vi "FlatToRichrfcontrol_CustomResponse.vi"(5 "OutputClusterType":T1, 11 "InputCluster":T2) -> (3 "OutputCluster":T1)   [LabVIEW 2024, in "FlexSDR_gRPC_client.lvlib"]
uses:
  FlexSDR_gRPC_client.lvlib
  rfcontrol_CustomResponse_Flat.ctl
  rfcontrol_CustomResponse.ctl
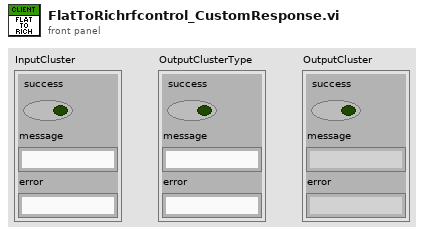
[diagram p1: front panel]
types:
  T1 = typedef "FlexSDR_gRPC_client.lvlib/rfcontrol_CustomResponse.ctl" = cluster{"success":bool, "message":string, "error":string}
  T2 = typedef "FlexSDR_gRPC_client.lvlib/rfcontrol_CustomResponse_Flat.ctl" = cluster{"success":bool, "message":string, "error":string}
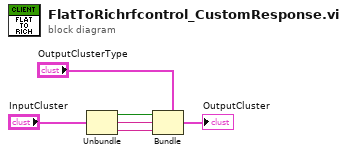
[diagram p0: block diagram]
diagram:
  n1 = Unbundle "Unbundle"("InputCluster") -> ("success"=w3:bool, "message"=w2:string, "error"=w1:string)
  n2 = Bundle "Bundle"(cluster="OutputClusterType", "success"=w3, "message"=w2, "error"=w1) -> (→"OutputCluster":T1)
